vi "Get Event Reg.vi"(8 "error in (no error)":errorcluster, 11 "Event in":refnum<class "Event.lvclass">) -> (0 "error out":errorcluster, 2 "Event Reg":refnum<event-registration>)   [LabVIEW 2022 SP3, in "Enclave.lvlib" / "Event.lvclass"]
uses:
  Event.lvclass
  Enclave Event.ctl
  Element.ctl
  Event.lvclass/Event.ctl
  Enclave.lvlib
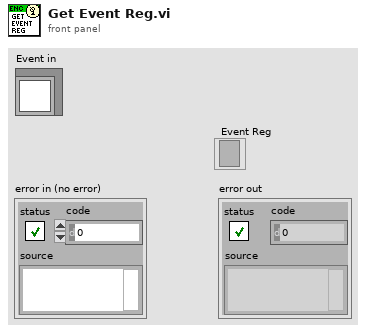
[diagram p1: front panel]
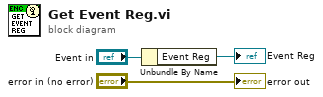
[diagram p0: block diagram]
diagram:
  n1 = Unbundle By Name("Event in") -> ("Event Reg"=→"Event Reg":refnum<event-registration>)
  "error out" <- "error in (no error)"
